vi "Time_seq.vi"() -> ()   [LabVIEW 2019]
uses:
  <vilib>/Platform/TimedLoop/XDataNode/timing_clust.ctl
  <vilib>/Platform/TimedLoop/XDataNode/nitl_modes.ctl
  <vilib>/Platform/TimedLoop/XDataNode/wakeup.ctl
  <vilib>/Platform/TimedLoop/XDataNode/XDataNode.xnode
  <vilib>/Platform/TimedLoop/XDataNode/XDNodeRunTimeDep.lvlib
panel:
  in  "Czas odniesienia":bool
  out "SpóŸnione wykonanie \ndrugiej ramki":bool
  out "?":bool
  out "?":bool
  out "?":bool
  in  "Start 3. ramki po 2. [s]":sgl min=0 step=0.2 format="%.1f"
  in  "Start 2. ramki po 1. [s]":sgl min=0 step=0.2 format="%.1f"
  out "?":bool
  out "?":bool
  out "?":bool
  in  "STOP":bool
  out "Start 3. ramki [s]":dbl format="%.3f"
  out "Start 2. ramki [s]":dbl format="%.3f"
  out "Start pierwszej ramki [ms]":dbl caption="Start 1. ramki [s]" format="%.3f"
  out "Komunikat\no b酬dzie":T1
  in  "Trwanie 3. ramki [s]":dbl=1.0 caption="Delay Time (s)" min=0.0 step=0.2
  in  "Trwanie 2. ramki [s]":dbl=1.0 caption="Delay Time (s)" min=0.0 step=0.2
  in  "Trwanie 1. ramki [s]":dbl=1.0 caption="Delay Time (s)" min=0.0 step=0.2
  # "Czasy zadane"
  # "Czasy zmierzone"
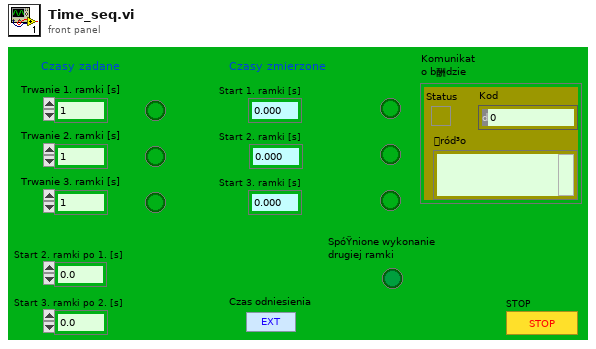
[diagram p1: front panel]
types:
  T1 = cluster{"Status":bool, "Kod":i32, "ród³o":string}
  T2 = typedef "XDNodeRunTimeDep.lvlib/timing_clust.ctl" = cluster{"Expected End [f-1]":u64, "Actual End [f-1]":u64, "Finished Late? [f-1]":bool, "Expected End [i-1]":u64, "Actual End [i-1]":u64, "Finished Late? [i-1]":bool, "Expected Start [i]":u64, "Actual Start [i]":u64, "Expected Start [f]":u64, "Actual Start [f]":u64, "Source Name":string, "Structure Name":string, "Period":i64, "Deadline":i64, "Offset":i64, "Start":i64, "Priority":i32, "Timeout":i32, "Mode":T3, "Wakeup Reason":T4, "Error":errorcluster, "Source Type":string, "Secondary Source Type":string, "Global End Time":u64, "Global Start Time":u64, "Frame Duration":u64, "Iteration Duration":u64, "Assigned CPU":i32, "I/O Scan Engine Mode":u32}
  T3 = typedef "XDNodeRunTimeDep.lvlib/nitl_modes.ctl" = enum32{"No Change", "Process missed periods, maintain original phase", "Discard missed periods, maintain original phase", "Process missed periods, ignore original phase", "Discard missed periods, ignore original phase"}
  T4 = typedef "XDNodeRunTimeDep.lvlib/wakeup.ctl" = enum32{"Normal", "Aborted", "Asynchronous wakeup", "Timing source error", "Timed loop error", "Timeout"}
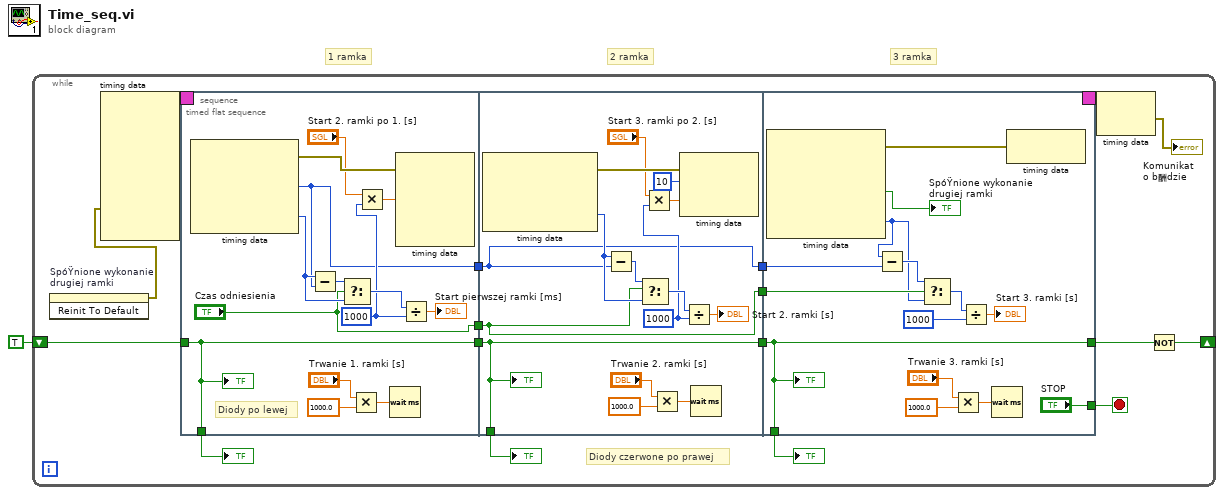
[diagram p0: block diagram]
diagram:
  # "3 ramka"
  # "2 ramka"
  # "1 ramka"
  n1 = while {
    shift-right: [w2] -> _
    shift-left: TRUE -> [w4]
    stop <- w6 stop-if-true
    # "Diody czerwone po prawej"
    n2 = invoke on="SpóŸnione wykonanie\ndrugiej ramki" class="Bool (strict)" method="Reinit To Default"() -> (error out=w5:errorcluster)  [unwired: 3 in, 2 out]
    n3 = node-c288(w5) -> (w12:T2)  [unwired: 7 in]
    n4 = timed-sequence {
      timing: w12 -> [_]
      timing-out: [_] -> w11
      tunnel: w4 -> [w24]
      tunnel: [w21] -> w9
      tunnel: [w20] -> w8
      tunnel: [w19] -> w7
      tunnel: [w18] -> w6
      tunnel: [w17] -> w3
      n5 = timed-flat-sequence {
        tunnel: w24 -> [w37]
        tunnel: [w37] -> w23
        tunnel: [w37] -> w21
        tunnel: ["Czas odniesienia"] -> w16
        tunnel: [w26] -> w14
        tunnel: w23 -> [w60]
        tunnel: [w60] -> w22
        tunnel: [w60] -> w20
        tunnel: w16 -> [w48]
        tunnel: [w48] -> w15
        tunnel: w14 -> [w47]
        tunnel: [w47] -> w13
        tunnel: w22 -> [w78]
        tunnel: [w78] -> w19
        tunnel: ["STOP"] -> w18
        tunnel: [w78] -> w17
        tunnel: w15 -> [w73]
        tunnel: w13 -> [w70]
        frame #0 {
          w27 = u16 1000 ("y")
          # "Diody po lewej"
          n6 = node-c288() -> (w38:errorcluster, w26:i64, w28:i64)  [unwired: 1 in, 2 out]
          n7 = Subtract(x=w28, y=w26) -> (x-y=w29:i64)
          n8 = Select(t=w29, s="Czas odniesienia", f=w28) -> (s? t:f=w30:i64)
          n9 = Multiply(x="Trwanie 1. ramki [s]", y=1000.0) -> (x*y=w33:dbl)
          n10 = Multiply(x="Start 2. ramki po 1. [s]", y=w27) -> (x*y=w35:sgl)
          n11 = Wait (ms)(milliseconds to wait=w33) -> ()  [unwired: 1 out]
          n12 = node-c288(w38, w35) -> ()  [unwired: 3 in, 1 out]
          n13 = Divide(x=w30, y=w27) -> (x/y=→"Start pierwszej ramki [ms]":dbl)
          "?" <- w37
        }
        frame #1 {
          w50 = u32 1000 ("y")
          n14 = node-c288() -> (w61:errorcluster, w49:i64)  [unwired: 1 in, 2 out]
          n15 = Subtract(x=w49, y=w47) -> (x-y=w52:i64)
          n16 = Select(t=w52, s=w48, f=w49) -> (s? t:f=w51:i64)
          n17 = Multiply(x="Start 3. ramki po 2. [s]", y=w50) -> (x*y=w57:sgl)
          n18 = Multiply(x="Trwanie 2. ramki [s]", y=1000.0) -> (x*y=w53:dbl)
          n19 = node-c288(w61, i64 10 ("Deadline"), w57) -> ()  [unwired: 1 out]
          n20 = Divide(x=w51, y=w50) -> (x/y=→"Start 2. ramki [s]":dbl)
          n21 = Wait (ms)(milliseconds to wait=w53) -> ()  [unwired: 1 out]
          "?" <- w60
        }
        frame #2 {
          n22 = node-c288() -> (w83:errorcluster, →"SpóŸnione wykonanie \ndrugiej ramki":bool, w71:i64)  [unwired: 1 in, 3 out]
          n23 = Subtract(x=w71, y=w70) -> (x-y=w72:i64)
          n24 = Select(t=w72, s=w73, f=w71) -> (s? t:f=w74:i64)
          n25 = Multiply(x="Trwanie 3. ramki [s]", y=1000.0) -> (x*y=w75:dbl)
          n26 = Divide(x=w74, y=u32 1000) -> (x/y=→"Start 3. ramki [s]":dbl)
          n27 = Wait (ms)(milliseconds to wait=w75) -> ()  [unwired: 1 out]
          n28 = node-c288(w83) -> ()  [unwired: 1 out]
          "?" <- w78
        }
      }
    }
    "?" <- w9
    "?" <- w8
    "?" <- w7
    n29 = node-c288(w11) -> (→"Komunikat\no b酬dzie":errorcluster)
    n30 = Not(x=w3) -> (.not. x?=w2:bool)
  }
